vi "Main.vi"   [LabVIEW 2015]
uses:
  <vilib>/NXT/Block Support/NXT_InputPort.ctl
  <vilib>/NXT/Subs/ColorSensorColors.ctl
  <vilib>/NXT/Block Support/NXT_OutputPort.ctl
  <vilib>/NXT/Dual Mode Library/Sensors/EV3_Color_Color.vi
  <vilib>/NXT/Dual Mode Library/Sensors/Touch_Released.vi
  <vilib>/NXT/Dual Mode Library/Sound/Tone.vi
  <vilib>/NXT/Dual Mode Library/Sensors/Read_NewTemp.vi
  <vilib>/NXT/NXTIO Xnodes/NXTIONodeSubVIs/NXTStopMotors.vi
  <vilib>/NXT/NXTIO Xnodes/NXTIONodeSubVIs/NXTMoveMotors.vi
  <vilib>/NXT/Dual Mode Library/Sensors/EV3_Color_Ambient.vi
  <vilib>/NXT/NXTIO Xnodes/AddressXNode/NXTIOAddress.xnode
  <vilib>/NXT/Subs/LVHSConnector.ctl
  <vilib>/NXT/NXTIO Xnodes/NXTIOXNode/NXTIO.xnode
  <vilib>/NXT/LegoClasses/BrickReference/BrickReference.lvclass
types:
  T1 = typedef "NXT_InputPort.ctl" = u32
  T2 = typedef "ColorSensorColors.ctl" = enum16{"No Color", "Black", "Blue", "Green", "Yellow", "Red", "White", "Brown"}
  T3 = typedef "NXT_OutputPort.ctl" = u8
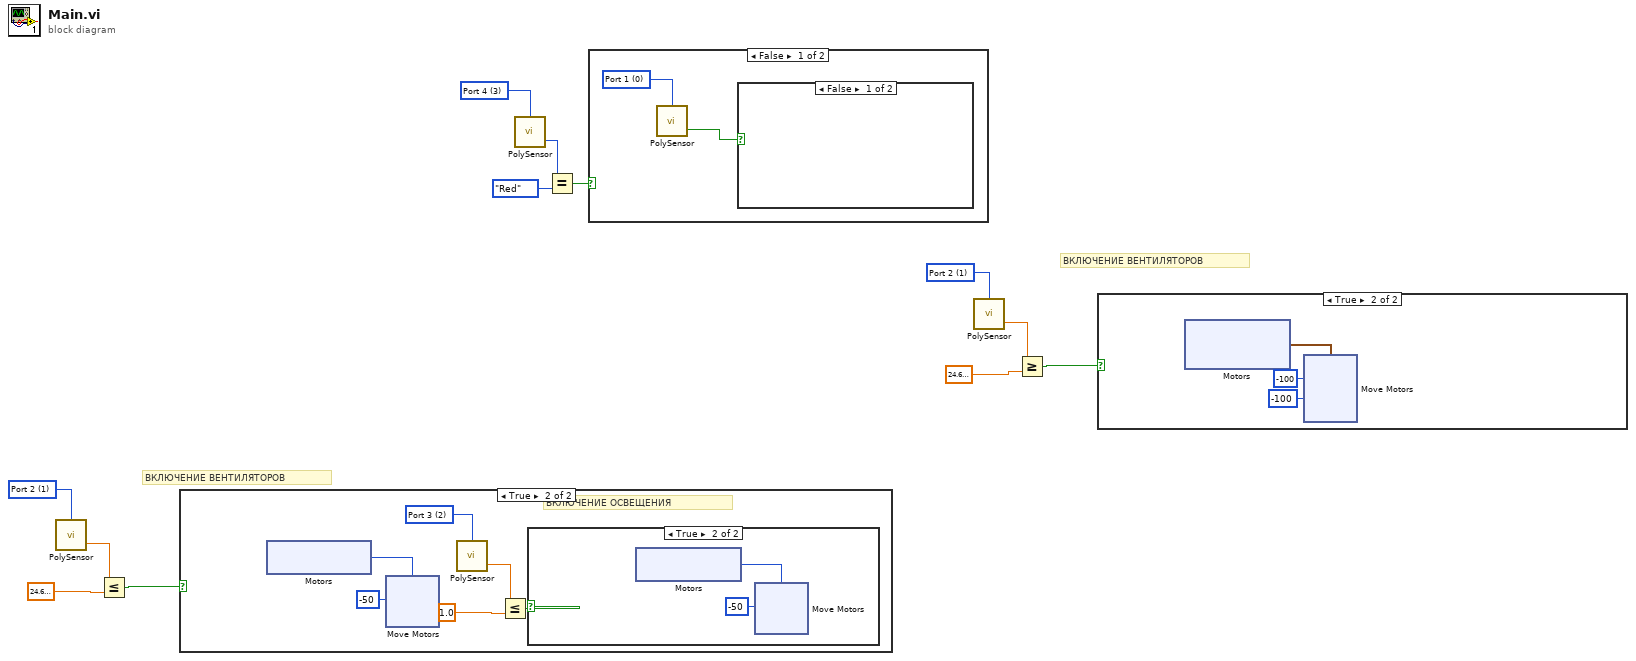
[diagram p0: block diagram]
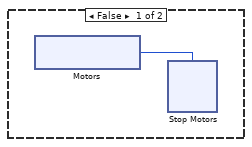
[diagram p2: hidden frame]
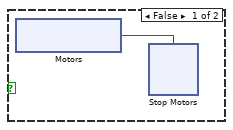
[diagram p3: hidden frame]
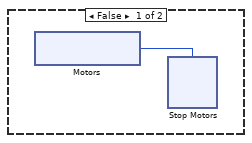
[diagram p4: hidden frame]
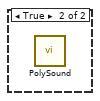
[diagram p5: hidden frame]
diagram:
  w1 = T1 1 items=["Port 1", "Port 2", "Port 3", "Port 4"] ("Port (Port 1)")
  w5 = T1 1 items=["Port 1", "Port 2", "Port 3", "Port 4"] ("Port (Port 1)")
  w12 = T1 3 items=["Port 1", "Port 2", "Port 3", "Port 4"] ("Port (Port 1)")
  # "ВКЛЮЧЕНИЕ ВЕНТИЛЯТОРОВ"
  # "ВКЛЮЧЕНИЕ ВЕНТИЛЯТОРОВ"
  n1 = call-poly <vilib>:"PolySensor.vi"("Port (Port 4)"=w1) -> ("Celsius"=w3:sgl)  [unwired: 2 in, 1 out]
  n2 = Less Or Equal?(x=w3, y=sgl 24.6) -> (x <= y?=w4:bool)
  n3 = case shown="True" w4 {
    frame False {
      n4 = xnode "Motors"() -> ("Motor"=w13:T3)
      n5 = xnode "Stop Motors"("Motors"=w13) -> ()  [unwired: 1 in, 1 out]
    }
    frame True {
      w23 = T1 2 items=["Port 1", "Port 2", "Port 3", "Port 4"] ("Port (Port 1)")
      # "ВКЛЮЧЕНИЕ ОСВЕЩЕНИЯ"
      n6 = xnode "Motors"() -> ("Motor"=w25:T3)
      n7 = xnode "Move Motors"("Power/Speed 1"=i8 -50, "Motors"=w25) -> ()  [unwired: 1 in, 1 out]
      n8 = call-poly <vilib>:"PolySensor.vi"("Port (Port 1)"=w23) -> ("Scaled Value"=w21:sgl)  [unwired: 2 in, 1 out]
      n9 = Less Or Equal?(x=w21, y=sgl 1.0) -> (x <= y?=w20:bool)
      n10 = case shown="True" w20 {
        frame False {
          n11 = xnode "Motors"() -> ("Motor"=w26:T3)
          n12 = xnode "Stop Motors"("Motors"=w26) -> ()  [unwired: 1 in, 1 out]
        }
        frame True {
          n13 = xnode "Motors"() -> ("Motor"=w33:T3)
          n14 = xnode "Move Motors"("Power/Speed 1"=i8 -50, "Motors"=w33) -> ()  [unwired: 1 in, 1 out]
        }
      }
    }
  }
  n15 = call-poly <vilib>:"PolySensor.vi"("Port (Port 1)"=w12) -> ("Detected Color"=w10:T2)  [unwired: 2 in, 1 out]
  n16 = Equal?(x=w10, y=ColorSensorColors."Red") -> (x = y?=w11:bool)
  n17 = case shown="False" w11 {
    frame False {
      w51 = T1 0 items=["Port 1", "Port 2", "Port 3", "Port 4"] ("Port (Port 1)")
      n18 = call-poly <vilib>:"PolySensor.vi"("Port (Port 1)"=w51) -> ("Yes / No"=w52:bool)  [unwired: 2 in, 1 out]
      n19 = case shown="False" w52 {
        frame False {
        }
        frame True {
          n20 = call-poly <vilib>:"PolySound.vi"() -> ()  [unwired: 4 in, 1 out]
        }
      }
    }
    frame True {
    }
  }
  n21 = call-poly <vilib>:"PolySensor.vi"("Port (Port 4)"=w5) -> ("Celsius"=w7:sgl)  [unwired: 2 in, 1 out]
  n22 = Greater Or Equal?(x=w7, y=sgl 24.6) -> (x >= y?=w8:bool)
  n23 = case shown="True" w8 {
    frame False {
      n24 = xnode "Motors"() -> ("Motor"=w53:T3)
      n25 = xnode "Stop Motors"("Motors"=w53) -> ()  [unwired: 1 in, 1 out]
    }
    frame True {
      n26 = xnode "Motors"() -> ("Motor"=w62:cluster{"Port":T3, "Port":T3})
      n27 = xnode "Move Motors"("Power/Speed 2"=i8 -100, "Power/Speed 1"=i8 -100, "Motors"=w62) -> ()  [unwired: 1 in, 1 out]
    }
  }
